vi "Init App Watcher.vi"(8 "error in (no error)":errorcluster, 11 "picoG in":refnum<class "picoG.lvclass">) -> (0 "error out":errorcluster, 3 "picoG out":refnum<class "picoG.lvclass">)   [LabVIEW 2020, in "PicoG-App.lvlib" / "picoG.lvclass"]
uses:
  picoG.lvclass
  picoG.lvclass/picoG.ctl
  App Watcher/App Watcher.lvclass
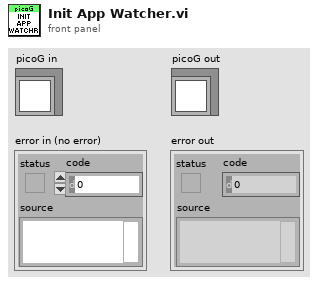
[diagram p1: front panel]
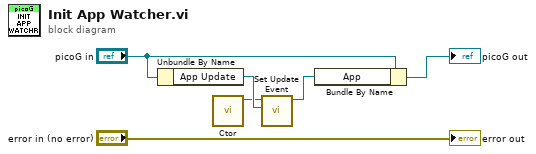
[diagram p0: block diagram]
diagram:
  n1 = Unbundle By Name("picoG in") -> ("App Update"=w3:refnum<user-event>)
  n2 = call "Ctor.vi"() -> ("App Watcher out"=w2:refnum<class "App Watcher.lvclass">)  [unwired: 10 in, 1 out]
  n3 = call "Set Update Event.vi"("App Update Event"=w3, "App Watcher in"=w2) -> ("App Watcher out"=w1:refnum<class "App Watcher.lvclass">)  [unwired: 8 in, 1 out]
  n4 = Bundle By Name(cluster="picoG in", "App"=w1) -> (→"picoG out":refnum<class "picoG.lvclass">)
  "error out" <- "error in (no error)"
